vi "PathPlanner_Path_PreCalcValues.vi"(11 "PathPlannerPath":T1={"BezierPoints"=[], "PreviewStartingRotation"={"VALUE"=0.0, "COS"=1.0, "SIN"=0.0}, "Reversed"=FALSE, "RotationTargets"=[], "ConstraintZones"=[], "EventMarkers"=[], "GlobalConstraints"={"MaxVelocityMps;"=0.0, "MaxAccelerationMpsSq;"=0.0, "MaxAngularVelRadPsEc;"=0.0, "MaxAngularAccRadPSecSq"=0.0, "Exists"=FALSE}, "GoalEndState"={"Velocity"=0.0, "Rotation"={"VALUE"=0.0, "COS"=1.0, "SIN"=0.0}}, "AllPoints"=[]} {"AllPoints"."HolonomicRotation"."SIN" format="%13.4f"; "AllPoints"."HolonomicRotation"."COS" format="%13.4f"; "AllPoints"."HolonomicRotation"."VALUE" format="%13.4f"; "AllPoints"."Position"."Y" format="%14.3f"; "AllPoints"."Position"."X" format="%14.3f"; "GoalEndState"."Rotation"."SIN" format="%13.4f"; "GoalEndState"."Rotation"."COS" format="%13.4f"; "GoalEndState"."Rotation"."VALUE" format="%13.4f"; "EventMarkers"."lastRobotPos"."Y" format="%14.3f"; "EventMarkers"."lastRobotPos"."X" format="%14.3f"; "EventMarkers"."markerPos"."Y" format="%14.3f"; "EventMarkers"."markerPos"."X" format="%14.3f"; "RotationTargets"."target"."SIN" format="%13.4f"; "RotationTargets"."target"."COS" format="%13.4f"; "RotationTargets"."target"."VALUE" format="%13.4f"; "PreviewStartingRotation"."SIN" format="%13.4f"; "PreviewStartingRotation"."COS" format="%13.4f"; "PreviewStartingRotation"."VALUE" format="%13.4f"; "BezierPoints"."Y" format="%14.3f"; "BezierPoints"."X" format="%14.3f"}) -> (3 "out PathPlannerPath":T1={"BezierPoints"=[], "PreviewStartingRotation"={"VALUE"=0.0, "COS"=1.0, "SIN"=0.0}, "Reversed"=FALSE, "RotationTargets"=[], "ConstraintZones"=[], "EventMarkers"=[], "GlobalConstraints"={"MaxVelocityMps;"=0.0, "MaxAccelerationMpsSq;"=0.0, "MaxAngularVelRadPsEc;"=0.0, "MaxAngularAccRadPSecSq"=0.0, "Exists"=FALSE}, "GoalEndState"={"Velocity"=0.0, "Rotation"={"VALUE"=0.0, "COS"=1.0, "SIN"=0.0}}, "AllPoints"=[]} {"AllPoints"."HolonomicRotation"."SIN" format="%13.4f"; "AllPoints"."HolonomicRotation"."COS" format="%13.4f"; "AllPoints"."HolonomicRotation"."VALUE" format="%13.4f"; "AllPoints"."Position"."Y" format="%14.3f"; "AllPoints"."Position"."X" format="%14.3f"; "GoalEndState"."Rotation"."SIN" format="%13.4f"; "GoalEndState"."Rotation"."COS" format="%13.4f"; "GoalEndState"."Rotation"."VALUE" format="%13.4f"; "EventMarkers"."lastRobotPos"."Y" format="%14.3f"; "EventMarkers"."lastRobotPos"."X" format="%14.3f"; "EventMarkers"."markerPos"."Y" format="%14.3f"; "EventMarkers"."markerPos"."X" format="%14.3f"; "RotationTargets"."target"."SIN" format="%13.4f"; "RotationTargets"."target"."COS" format="%13.4f"; "RotationTargets"."target"."VALUE" format="%13.4f"; "PreviewStartingRotation"."SIN" format="%13.4f"; "PreviewStartingRotation"."COS" format="%13.4f"; "PreviewStartingRotation"."VALUE" format="%13.4f"; "BezierPoints"."Y" format="%14.3f"; "BezierPoints"."X" format="%14.3f"})   [LabVIEW 2019, in "PathPlanner24.lvlib"]
uses:
  PathPlanner24.lvlib
  TypeDef/PathPlannerPath.ctl
  <vilib>/Rock Robotics/WPI/ThirdParty/JAS_Junk/TrajLib/TypeDef/TRANSLATION2D.ctl
  <vilib>/Rock Robotics/WPI/ThirdParty/JAS_Junk/TrajLib/TypeDef/ROTATION2D.ctl
  TypeDef/PathPlannerRotationTarget.ctl
  TypeDef/PathPlannerConstraintsZone.ctl
  TypeDef/PathPlannerPathConstraints.ctl
  TypeDef/PathPlannerEventMarker.ctl
  TypeDef/PathPlannerCommand.ctl
  TypeDef/PathPlannerGoalEndState.ctl
  TypeDef/PathPlannerPathPoint.ctl
  <vilib>/Rock Robotics/WPI/ThirdParty/JAS_Junk/TrajLib/Util_CalcDist.vi
  PathPlanner_GeomUtil_CalculateRadius.vi
  <vilib>/Rock Robotics/WPI/ThirdParty/JAS_Junk/TrajLib/Translation2d_Minus.vi
  <vilib>/Rock Robotics/WPI/ThirdParty/JAS_Junk/TrajLib/Translation2d_GetXY.vi
  <vilib>/Rock Robotics/WPI/ThirdParty/JAS_Junk/TrajLib/Translation2d_Create.vi
  <vilib>/Rock Robotics/WPI/ThirdParty/JAS_Junk/TrajLib/Trajectory_Library.lvlib
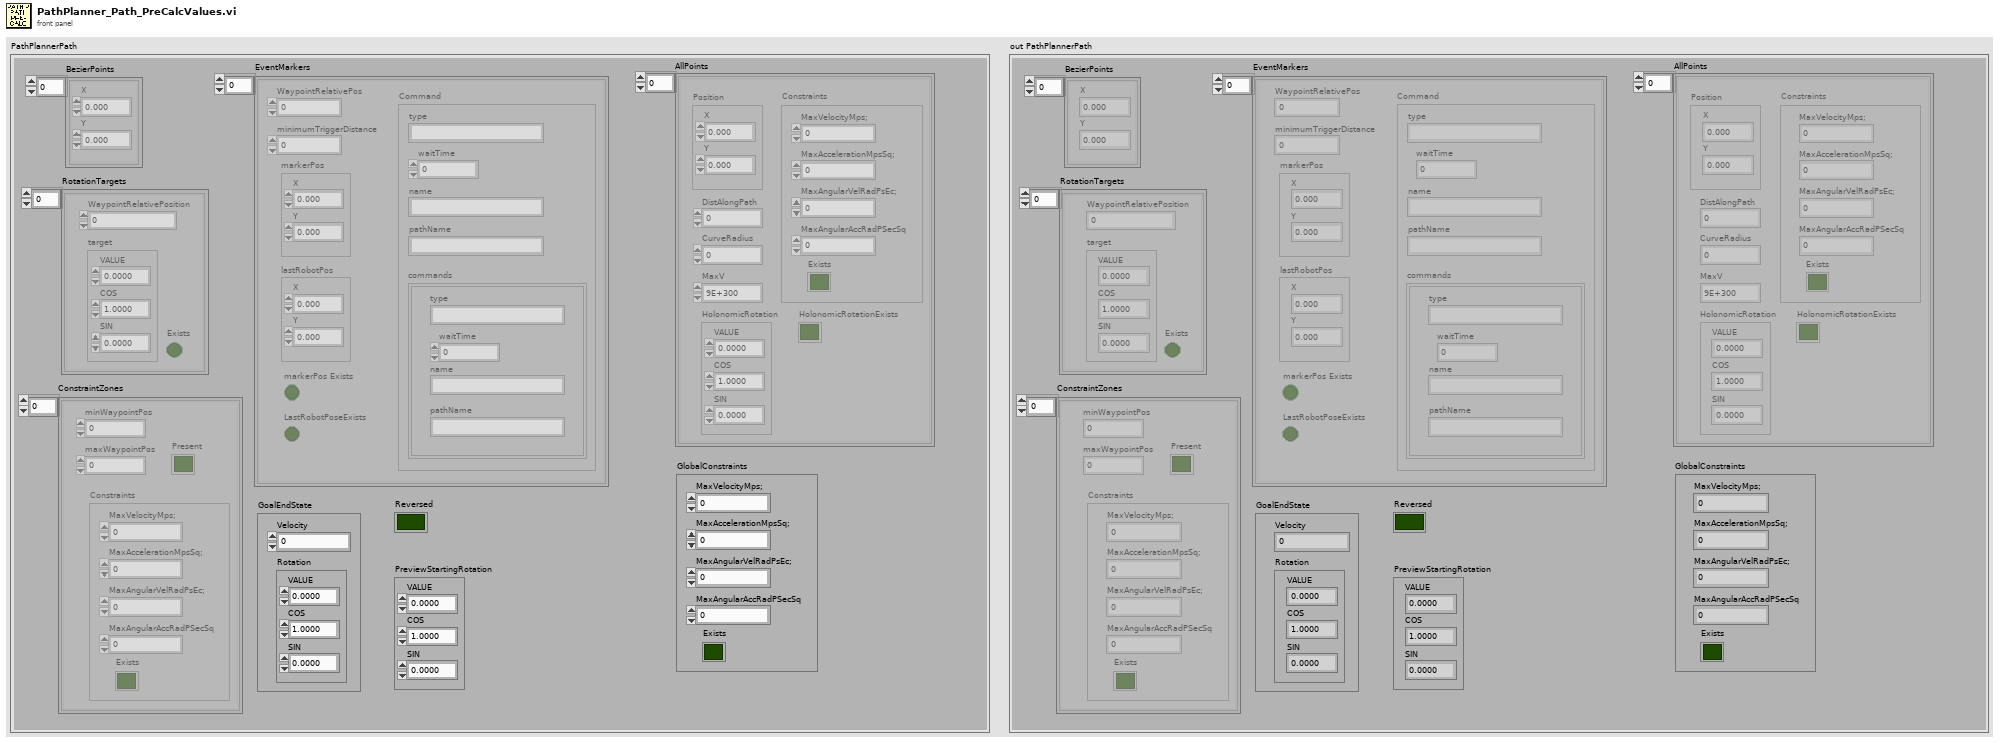
[diagram p1: front panel]
types:
  T1 = typedef "PathPlanner24.lvlib/PathPlannerPath.ctl" = cluster{"BezierPoints":T2[], "PreviewStartingRotation":T3, "Reversed":bool, "RotationTargets":T4[], "ConstraintZones":T5[], "EventMarkers":T7[], "GlobalConstraints":T6, "GoalEndState":T9, "AllPoints":T10[]}
  T2 = typedef "Trajectory_Library.lvlib/TRANSLATION2D.ctl" = cluster{"X":dbl, "Y":dbl}
  T3 = typedef "Trajectory_Library.lvlib/ROTATION2D.ctl" = cluster{"VALUE":dbl, "COS":dbl, "SIN":dbl}
  T4 = typedef "PathPlanner24.lvlib/PathPlannerRotationTarget.ctl" = cluster{"target":T3, "WaypointRelativePosition":dbl, "Exists":bool}
  T5 = typedef "PathPlanner24.lvlib/PathPlannerConstraintsZone.ctl" = cluster{"minWaypointPos":dbl, "maxWaypointPos":dbl, "Constraints":T6, "Present":bool}
  T6 = typedef "PathPlanner24.lvlib/PathPlannerPathConstraints.ctl" = cluster{"MaxVelocityMps;":dbl, "MaxAccelerationMpsSq;":dbl, "MaxAngularVelRadPsEc;":dbl, "MaxAngularAccRadPSecSq":dbl, "Exists":bool}
  T7 = typedef "PathPlanner24.lvlib/PathPlannerEventMarker.ctl" = cluster{"WaypointRelativePos":dbl, "minimumTriggerDistance":dbl, "markerPos":T2, "lastRobotPos":T2, "Command":T8, "markerPos Exists":bool, "LastRobotPoseExists":bool}
  T8 = typedef "PathPlanner24.lvlib/PathPlannerCommand.ctl" = cluster{"waitTime":dbl, "name":string, "type":string, "pathName":string, "commands":cluster{"type":string, "waitTime":dbl, "name":string, "pathName":string}[]}
  T9 = typedef "PathPlanner24.lvlib/PathPlannerGoalEndState.ctl" = cluster{"Velocity":dbl, "Rotation":T3}
  T10 = typedef "PathPlanner24.lvlib/PathPlannerPathPoint.ctl" = cluster{"Position":T2, "HolonomicRotation":T3, "DistAlongPath":dbl, "CurveRadius":dbl, "MaxV":dbl, "Constraints":T6, "HolonomicRotationExists":bool}
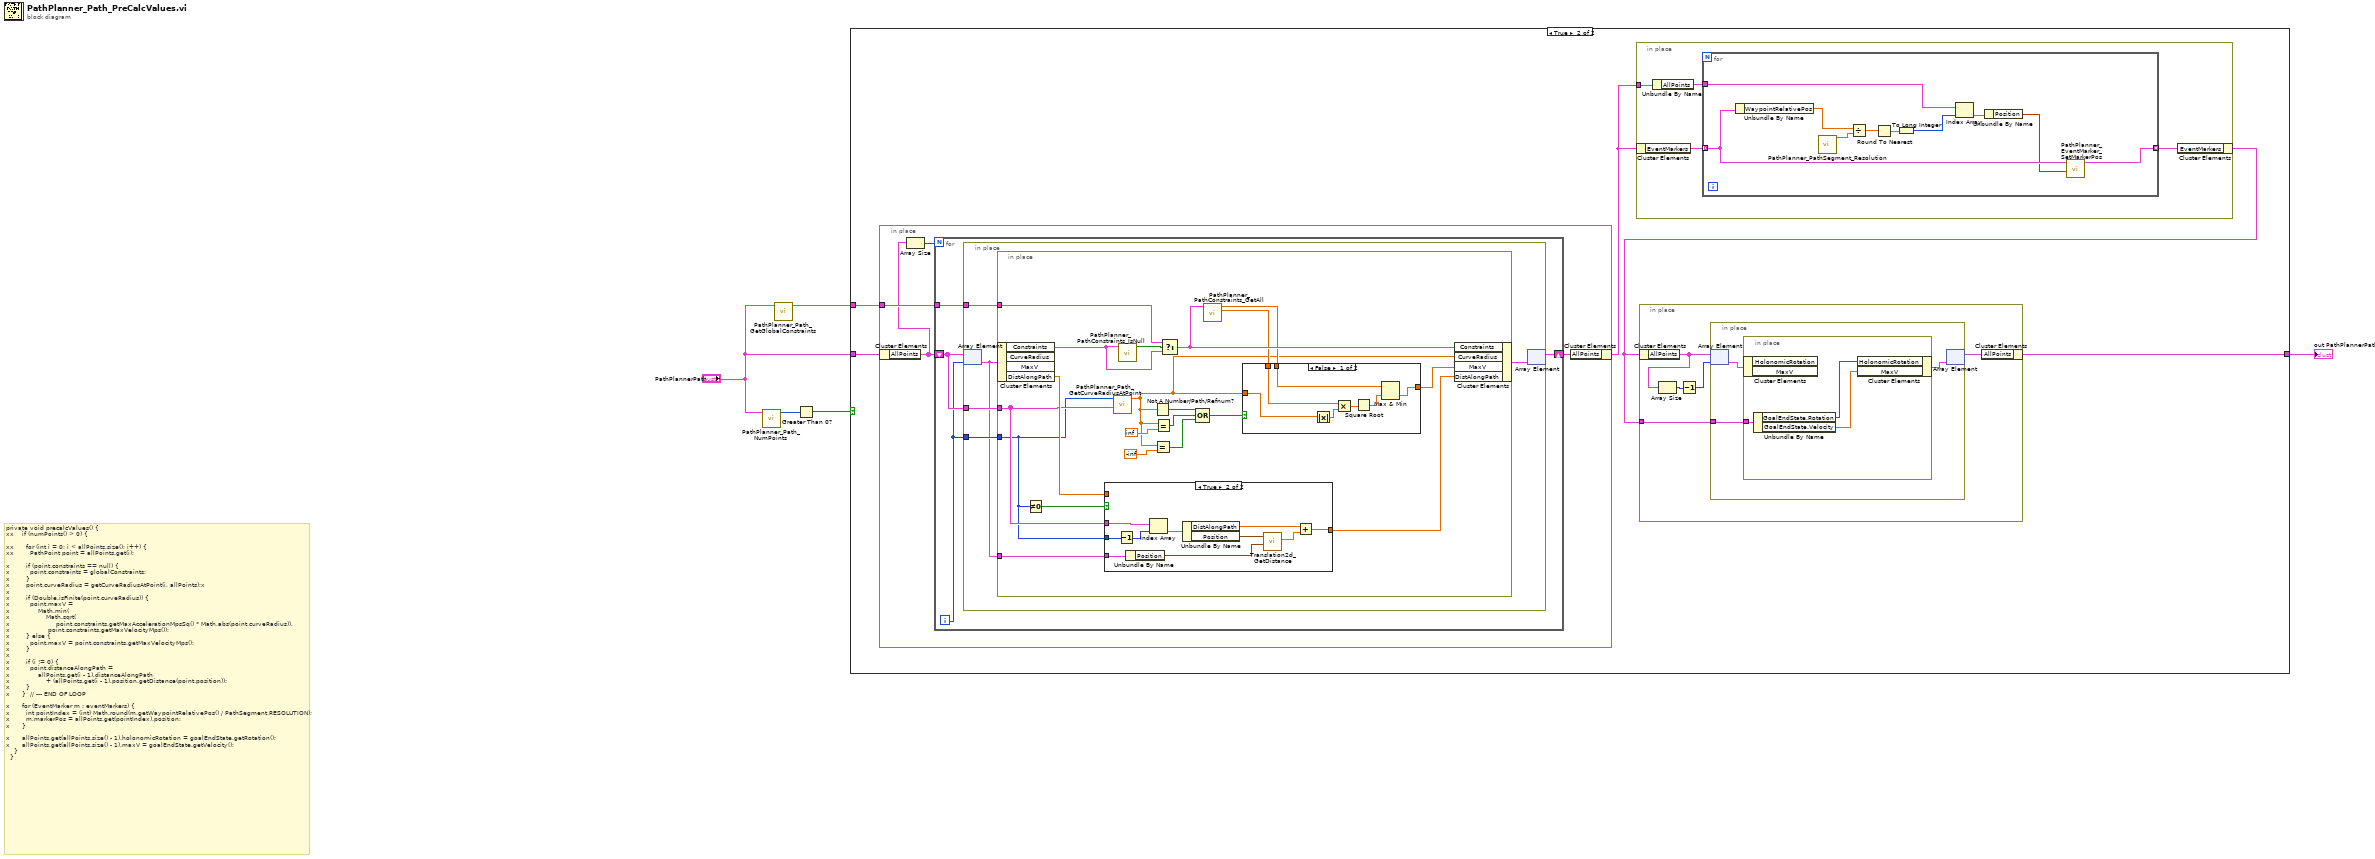
[diagram p0: block diagram]
diagram:
  # "private void precalcValues() {\nxx    if (numPoints() > 0) {\n\nxx      for (int i = 0; i < allPoints.size(); i++) {\nxx        PathPoint point = allPoints.get(i);\n\nx        if (point.constraints == null) {\nx          point.constraints = globalConstraints;\nx        }\nx        point.curveRadius = getCurveRadiusAtPoint(i, allPoints);x\nx\nx        if (Double.isFinite(point.curveRadius)) {\nx          point.maxV =\nx              Math.min(\nx                  Math.sqrt(\nx                      \tpoint.constraints.getMaxAccelerationMpsSq() * Math.abs(point.curveRadius)),\nx                  \tpoint.constraints.getMaxVelocityMps());\nx        } else {\nx          point.maxV = point.constraints.getMaxVelocityMps();\nx        }\nx\nx        if (i != 0) {\nx          point.distanceAlongPath =\nx              allPoints.get(i - 1).distanceAlongPath\nx                  + (allPoints.get(i - 1).position.getDistance(point.position));\nx        }\nx      }  // --- END OF LOOP\n\nx      for (EventMarker m : eventMarkers) {\nx        int pointIndex = (int) Math.round(m.getWaypointRelativePos() / PathSegment.RESOLUTION);\nx        m.markerPos = allPoints.get(pointIndex).position;\nx      }\n\nx      allPoints.get(allPoints.size() - 1).holonomicRotation = goalEndState.getRotation();\nx      allPoints.get(allPoints.size() - 1).maxV = goalEndState.getVelocity();\n    }\n  }"
  n1 = call "PathPlanner_Path_NumPoints.vi"("PathPlannerPath"="PathPlannerPath") -> ("NumPoints"=w5:i32)  [unwired: 10 in]
  n2 = call "PathPlanner_Path_GetGlobalConstraints.vi"("PathPlannerPath"="PathPlannerPath") -> ("GlobalConstraints"=w1:T6)  [unwired: 10 in]
  n3 = Greater Than 0?(x=w5) -> (x > 0?=w4:bool)
  n4 = case shown="True" w4 {
    tunnel: "PathPlannerPath" -> [w6 w11]
    tunnel: [w6 w9] -> w3
    tunnel: w1 -> [_ w10]
    frame False {
    }
    frame True {
      n5 = in-place {
        in-place-border: w10 -> [w40]
        n6 = in-place-cluster #1(w11) -> ("AllPoints"=w38:T10[])
        n7 = Array Size(array=w38) -> (size(s)=w39:i32)
        n8 = for {
          N: w39 -> [_]
          tunnel: w40 -> [w44]
          shift-right: [w41] -> w37
          shift-left: w38 -> [w43]
          i -> [w42]
          n9 = in-place {
            in-place-border: w44 -> [w48]
            in-place-border: w43 -> [w47]
            in-place-border: w42 -> [w46]
            n10 = in-place-array #2(w43, w42) -> (w45:T10)
            n11 = in-place {
              in-place-border: w48 -> [w67]
              in-place-border: w47 -> [w55]
              in-place-border: w46 -> [w54]
              in-place-border: w45 -> [w53]
              n12 = in-place-cluster #3(w45) -> ("Constraints"=w68:T6, "DistAlongPath"=w57:dbl)  [unwired: 2 out]
              n13 = Not Equal To 0?(x=w54) -> (x != 0?=w58:bool)
              n14 = case shown="True" w58 {
                tunnel: w57 -> [w70 _]
                tunnel: [w70 w71] -> w56
                tunnel: w55 -> [_ w80]
                tunnel: w54 -> [_ w78]
                tunnel: w53 -> [_ w75]
                frame False {
                }
                frame True {
                  n15 = Decrement(x=w78) -> (x-1=w79:i32)
                  n16 = Unbundle By Name(w75) -> ("Position"=w74:T2)
                  n17 = Index Array(array=w80, index=w79) -> (element=w77:T10)
                  n18 = Unbundle By Name(w77) -> ("DistAlongPath"=w73:dbl, "Position"=w76:T2)
                  n19 = call <vilib>:"Translation2d_GetDistance.vi"("other Translation"=w74, "In Translation"=w76) -> ("Distance"=w72:dbl)  [unwired: 9 in]
                  n20 = Add(x=w73, y=w72) -> (x+y=w71:dbl)
                }
              }
              n21 = call "PathPlanner_Path_GetCurveRadiusAtPoint.vi"("Points"=w55, "Index"=w54) -> ("Radius"=w51:dbl)  [unwired: 9 in]
              n22 = call "PathPlanner_PathConstraints_IsNull.vi"("PathPlannerConstraints"=w68) -> ("IsNull"=w69:bool)  [unwired: 10 in]
              n23 = Not A Number/Path/Refnum?(number/path/refnum=w51) -> (NaN/Path/Refnum?=w63:bool)
              n24 = Equal?(x=w51, y=-inf) -> (x = y?=w50:bool)
              n25 = Equal?(x=w51, y=inf) -> (x = y?=w62:bool)
              n26 = Select(t=w67, s=w69, f=w68) -> (s? t:f=w66:T6)
              n27 = Compound Arithmetic op=OR(w63, w62, w50) -> (w60:bool)
              n28 = call "PathPlanner_PathConstraints_GetAll.vi"("PathPlannerConstraints"=w66) -> ("MaxAccelerationMpsSq;"=w59:dbl, "MaxVelocityMps;"=w65:dbl)  [unwired: 6 in, 3 out]
              n29 = case shown="False" w60 {
                tunnel: w65 -> [w86 w88]
                tunnel: [w87 w88] -> w64
                tunnel: w59 -> [w83 _]
                tunnel: w51 -> [w81 _]
                frame False {
                  n30 = Absolute Value(x=w81) -> (abs(x)=w84:dbl)
                  n31 = Multiply(x=w83, y=w84) -> (x*y=w82:dbl)
                  n32 = Square Root(x=w82) -> (sqrt(x)=w85:dbl)
                  n33 = Max & Min(x=w86, y=w85) -> (min(x,y)=w87:dbl)  [unwired: 1 out]
                }
                frame True {
                }
              }
              n34 = in-place-cluster #3("Constraints"=w66, "CurveRadius"=w51, "MaxV"=w64, "DistAlongPath"=w56) -> (w49:T10)
            }
            n35 = in-place-array #2(w49) -> (w41:T10[])  [unwired: 1 out]
          }
        }
        n36 = in-place-cluster #1("AllPoints"=w37) -> (w7:T1)
      }
      n37 = in-place {
        in-place-border: w7 -> [w13]
        n38 = in-place-cluster #4(w7) -> ("EventMarkers"=w15:T7[])
        n39 = Unbundle By Name(w13) -> ("AllPoints"=w12:T10[])
        n40 = for {
          tunnel: w15 -> [w18] mode=indexing
          tunnel: [w16] -> w14 mode=indexing
          tunnel: w12 -> [w25]
          n41 = Unbundle By Name(w18) -> ("WaypointRelativePos"=w21:dbl)
          n42 = call "PathPlanner_PathSegment_Resolution.vi"() -> ("Resolution"=w24:dbl)  [unwired: 11 in]
          n43 = Divide(x=w21, y=w24) -> (x/y=w23:dbl)
          n44 = Round To Nearest(number=w23) -> (nearest integer value=w22:dbl)
          n45 = To Long Integer(number=w22) -> (32bit integer=w20:i32)
          n46 = Index Array(array=w25, index=w20) -> (element=w19:T10)
          n47 = Unbundle By Name(w19) -> ("Position"=w17:T2)
          n48 = call "PathPlanner_EventMarker_SetMarkerPos.vi"("MarkerPos"=w17, "in EventMarker"=w18) -> ("out EventMarker"=w16:T7)  [unwired: 9 in]
        }
        n49 = in-place-cluster #4("EventMarkers"=w14) -> (w8:T1)
      }
      n50 = in-place {
        in-place-border: w8 -> [w26]
        n51 = in-place-cluster #5(w8) -> ("AllPoints"=w29:T10[])
        n52 = Array Size(array=w29) -> (size(s)=w30:i32)
        n53 = Decrement(x=w30) -> (x-1=w28:i32)
        n54 = in-place {
          in-place-border: w26 -> [w31]
          n55 = in-place-array #6(w29, w28) -> (w33:T10)
          n56 = in-place {
            in-place-border: w31 -> [w36]
            n57 = in-place-cluster #7(w33) -> ()  [unwired: 2 out]
            n58 = Unbundle By Name(w36) -> ("GoalEndState.Rotation"=w35:T3, "GoalEndState.Velocity"=w34:dbl)
            n59 = in-place-cluster #7("HolonomicRotation"=w35, "MaxV"=w34) -> (w32:T10)
          }
          n60 = in-place-array #6(w32) -> (w27:T10[])  [unwired: 1 out]
        }
        n61 = in-place-cluster #5("AllPoints"=w27) -> (w9:T1)
      }
    }
  }
  "out PathPlannerPath" <- w3
